vi "Register for Events (Enum).vi"(8 "error in (no error)":errorcluster, 9 "VEnum of Object.Method names":variant, 11 "JKI_Python_Server in":refnum<class "Server.lvclass">) -> (0 "error out":errorcluster, 1 "Python Event":T1, 3 "JKI_Python_Server out":refnum<class "Server.lvclass">)   [LabVIEW 2013, in "JKI_Python_Bridge_for_LV.lvlib" / "Server.lvclass"]
uses:
  Server.lvclass
  PyObject/PyObject.lvclass
  Type Definitions/Public Events - Cluster.ctl
  Call/Call.lvclass
  Type Definitions/Python Method Call - Event Registration.ctl
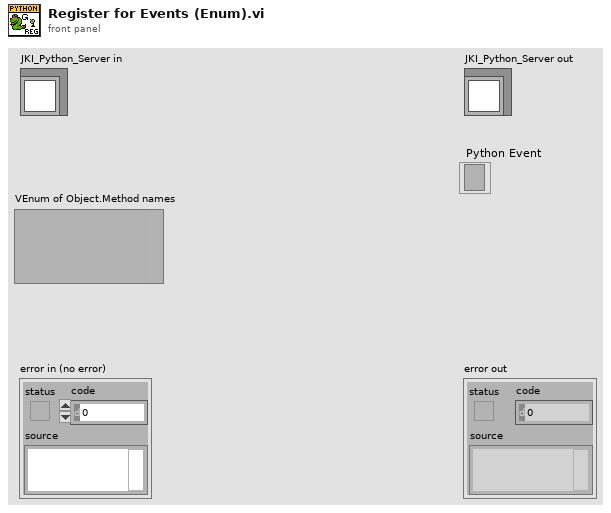
[diagram p1: front panel]
types:
  T1 = typedef "JKI_Python_Bridge_for_LV.lvlib/Server.lvclass/Python Method Call - Event Registration.ctl" = refnum<event-registration>
  T2 = typedef "Type Descriptor Enumeration__ogtk.ctl" = enum8{"<Null>", "I8", "I16", "I32", "I64", "U8", "U16", "U32", "U64", "SGL", "DBL", "EXT", "CSG", "CDB", "CXT", "0x0F", "0x10", "0x11", "0x12", "0x13", "0x14", "Enum U8", "Enum U16", "Enum U32", "Enum U64", "SGL PQ", "DBL PQ", "EXT PQ", "CSG PQ", "CDB PQ", "CXT PQ", "0x1F", "0x20", "Boolean", "0x22", "0x23", "0x24", "0x25", "0x26", "0x27", "0x28", "0x29", "0x2A", "0x2B", "0x2C", "0x2D", "0x2E", "0x2F", "String", "0x31", "Path", "Pict", "0x34", "0x35", "0x36", "DAQ", "0x38", "0x39", "0x3A", "0x3B", "0x3C", "0x3D", "0x3E", "0x3F", "Array", "0x41", "0x42", "0x43", "0x44", "0x45", "0x46", "0x47", "0x48", "0x49", "0x4A", "0x4B", "0x4C", "0x4D", "0x4E", "0x4F", "Cluster", "0x51", "0x52", "Variant", "Waveform", "0x55", "0x56", "0x57", "0x58", "0x59", "0x5A", "0x5B", "0x5C", "0x5D", "0x5E", "0x5F", "0x60", "0x61", "0x62", "0x63", "0x64", "0x65", "0x66", "0x67", "0x68", "0x69", "0x6A", "0x6B", "0x6C", "0x6D", "0x6E", "0x6F", "Refnum"}
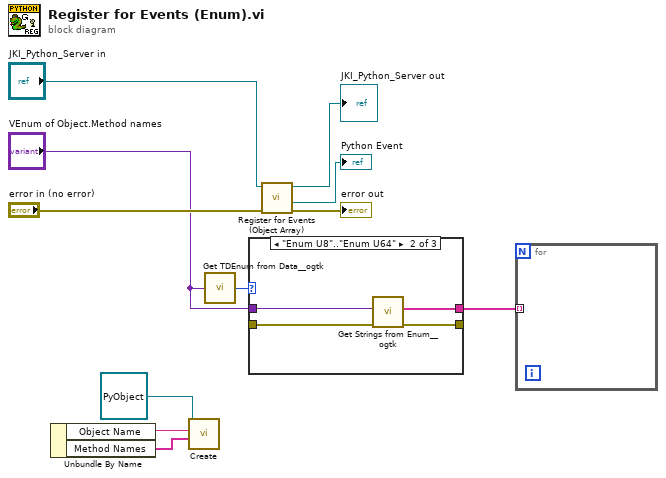
[diagram p0: block diagram]
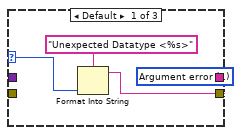
[diagram p2: hidden frame]
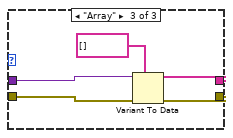
[diagram p3: hidden frame]
diagram:
  n1 = Unbundle By Name() -> ("Object Name"=w8:string, "Method Names"=w7:string[])  [unwired: 1 in]
  n2 = call "Create.vi"("Method Names"=w7, "Object Name"=w8, "Node in"=refnum<class "PyObject.lvclass"> refnum) -> ("error in (no error)"=w5:errorcluster)  [unwired: 6 in, 2 out]
  n3 = call <userlib>:"Get TDEnum from Data__ogtk.vi"("Data"="VEnum of Object.Method names") -> ("Type Descriptor Enumeration"=w4:T2)  [unwired: 4 in]
  n4 = case shown="\"Enum U8\"..\"Enum U64\"" w4 {
    selector: w4 -> [w14 _ _]
    tunnel: [_ w22 w27] -> w1
    tunnel: [w15 w21 w26] -> _
    tunnel: [_ w20 w25] -> w3
    tunnel: "VEnum of Object.Method names" -> [_ w19 w24]
    frame Default {
      w18 = 1 items=["No error", "Argument error", "Memory is full", "Out of zone", "End of file", "File already open", "Generic file I/O error", "File not found", "File permission error", "Disk is full", "Duplicate path", "Too many files open", "System feature not enabled", "Resource file not found", "Cannot add resource", "Resource not found", "Image not found", "Image memory error", "Pen does not exist", "Config type invalid", "Config token not found", "Config parse error", "Config memory error", "Bad external code format", "Bad external code offset", "External code not present", "Null window", "Destroy window error", "Null menu", "Print aborted", "Bad print record", "Print driver error", "Windows error during printing", "Memory error during printing", "Print dialog error", "Generic print error", "Invalid device refnum", "Device not found", "Device parameter error", "Device unit error", "Cannot open device", "Device call aborted", "Generic error", "Cancelled by user", "Object ID too low", "Object ID too high", "Object not in heap", "Unknown heap", "Unknown object (invalid DefProc)", "Unknown object (DefProc not in table)", "Message out of range", "Invalid (null) method", "Unknown message", "Manager call not supported", "Bad address", "Network operation in progress", "Network operation timed out", "Connection is busy", "Network attribute not supported", "Network error", "Address in use", "System out of memory", "Connection aborted", "Connection refused", "Not connected", "Already connected", "Connection closed", "Initialization error (interapplication manager)", "Bad occurrence", "Wait on unbound occurrence handler", "Occurrence queue overflow", "Datalog type conflict", "Unused", "Unrecognized type (interapplication manager)", "Memory corrupt", "Failed to make temporary DLL", "Old CIN version", "Drag socket not found", "Failed to load drop-object", "Failed to register OLE object", "Failed to release OLE object", "Format specifier type mismatch", "Unknown format specifier", "Too few format specifiers", "Too many format specifiers", "Scan failed", "Newer CIN version", "Error converting to variant", "Runtime menu error", "Password tampered", "Variant attribute not found", "Incompatible variant data type", "Event data is not available", "Event Store is not present", "Occurrence is not found", "Event Queue is not created", "Event info is not available", "Refnum passed is NULL", "Error retrieving Class GUID", "Error retrieving CoClass GUID", "Error retrieving TypeLib GUID.", "Bad built application magic bytes.", "Specific driver is different from the specific driver associated with the Logical Name.", "There is no session opened to the class driver.", "Max Error", "MAX - Error with config objects", "MAX - Error loading configuration", "MAX - Group not supported"]
      n5 = Format Into String(format string="Unexpected Datatype <%s>" ("Format String"), w14) -> (resulting string=w16:string)  [unwired: 2 in, 1 out]
      n6 = call <userlib>:"Build Error Cluster__ogtk.vi"("String to Prepend to source (\"\")"=w16, "code"=w18) -> ("error out"=w15:errorcluster)
    }
    frame "Enum U8".."Enum U64" {
      n7 = call <userlib>:"Get Strings from Enum__ogtk.vi"("error in (no error)"=w20, "Enum"=w19) -> ("error out"=w21:errorcluster, "Enum Strings"=w22:string[])  [unwired: 6 in, 2 out]
    }
    frame "Array" {
      n8 = Variant To Data(error in=w25, type=string[] [] ("Functions"), Variant=w24) -> (data=w27:string[], error out=w26:errorcluster)
    }
  }
  n9 = call "Register for Events (Object Array).vi"("error in (no error)"="error in (no error)", "JKI_Python_Server in"="JKI_Python_Server in") -> ("error out"=→"error out":errorcluster, "Python Event"=→"Python Event":T1, "JKI_Python_Server out"=→"JKI_Python_Server out":refnum<class "Server.lvclass">)  [unwired: 7 in]
  n10 = for {
    tunnel: w1 -> [_] mode=indexing
  }
